vi "Calibration Hot Limit (Set).vi"(6 "ISOBUS address":T4=-1 caption="ISOBUS address (-1)", 8 "error in":errorcluster, 9 "Unit":T1, 10 "Hot Limit":dbl min=-100.0 max=100.0 step=0.1, 11 "Mercury Reference In":T5) -> (0 "error out":errorcluster, 2 "Response":T2, 3 "Mercury Reference Out":T5, 4 "Valid?":T3)   [LabVIEW 2013, in "Mercury iXX.lvlib" / "Temperature.lvlib"]
doc: "Set the current calibration offset for the selected temperature device."
uses:
  Temperature.lvlib
  Mercury iXX.lvlib
  Private/Controls/Command Verbs.ctl
  Controls/Response String.ctl
  Controls/Is Valid LED.ctl
  Controls/Comms Transport Layer.ctl
  Controls/Mercury Reference.ctl
  Controls/ISOBus Address.ctl
  Private/Controls/Query Dynamic Reference.ctl
  Controls/Unit String.ctl
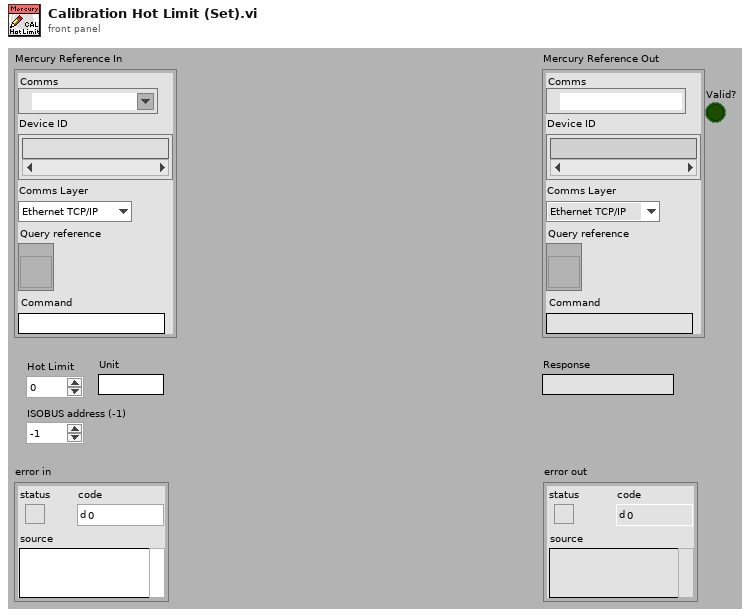
[diagram p1: front panel]
types:
  T1 = typedef "Mercury iXX.lvlib/Unit String.ctl" = string
  T2 = typedef "Mercury iXX.lvlib/Response String.ctl" = string
  T3 = typedef "Mercury iXX.lvlib/Is Valid LED.ctl" = bool
  T4 = typedef "Mercury iXX.lvlib/ISOBus Address.ctl" = i32
  T5 = typedef "Mercury iXX.lvlib/Mercury Reference.ctl" = cluster{"Comms":refnum<visa-resource-name>, "Device ID":string[], "Comms Layer":T6, "Command":string, "Query reference":T7}
  T6 = typedef "Mercury iXX.lvlib/Comms Transport Layer.ctl" = enum16{"Ethernet TCP/IP", "USB", "ISOBus - RS-232", "GPIB"}
  T7 = typedef "Mercury iXX.lvlib/Query Dynamic Reference.ctl" = refnum<vi>
  T8 = typedef "Mercury iXX.lvlib/Command Verbs.ctl" = string
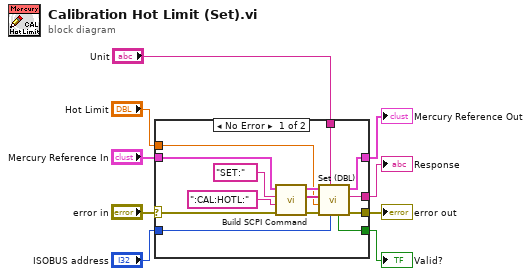
[diagram p0: block diagram]
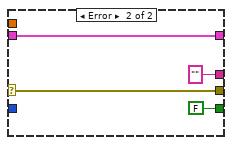
[diagram p2: hidden frame]
diagram:
  n1 = case shown="No Error" "error in" {
    selector: "error in" -> [w12 w27]
    tunnel: "Mercury Reference In" -> [w18 w26]
    tunnel: [w17 w26] -> w8
    tunnel: [w16 w27] -> w7
    tunnel: "ISOBUS address" -> [w15 _]
    tunnel: [w14 T3 FALSE ("Valid?")] -> w5
    tunnel: [w13 T2 "" ("Response")] -> w4
    tunnel: "Hot Limit" -> [w11 _]
    tunnel: "Unit" -> [w10 _]
    frame No Error {
      n2 = call "Build SCPI Command.vi"("error in"=w12, "Noun(s)"=":CAL:HOTL:" ("Command"), "Verb"=T8 "SET:", "Mercury Reference In"=w18) -> ("error out"=w20:errorcluster, "SCPI Message(s)"=w21:string[], "Mercury Reference Out"=w22:T5)  [unwired: 5 out]
      n3 = call "Set (DBL).vi"("ISOBUS address"=w15, "Unit"=w10, "error in"=w20, "Command Value (Dbl)"=w11, "SCPI Message(s)"=w21, "Mercury Reference In"=w22) -> ("error out"=w16:errorcluster, "Response"=w13:T2, "Mercury Reference Out"=w17:T5, "Valid?"=w14:T3)  [unwired: 2 out]
    }
    frame Error {
    }
  }
  "Mercury Reference Out" <- w8
  "error out" <- w7
  "Valid?" <- w5
  "Response" <- w4
